vi "workbook add format.vi"(8 "error in (no error)":errorcluster, 11 "workbook":u32) -> (0 "error out":errorcluster, 3 "function return":u32)   [LabVIEW 8.6]
doc: "lxw_format workbook_add_format(lxw_workbook workbook);"
uses:
  pending_lvxlsxwriter/xlsxwriter.dll
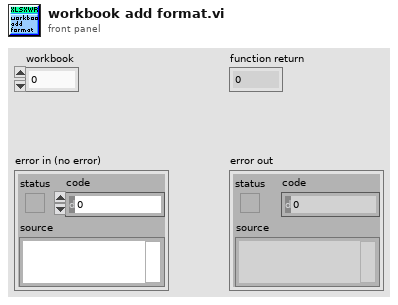
[diagram p1: front panel]
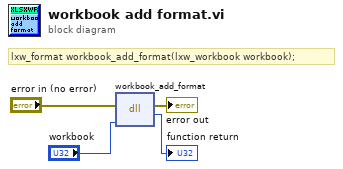
[diagram p0: block diagram]
diagram:
  # "lxw_format workbook_add_format(lxw_workbook workbook);"
  n1 = dll-call lib="C:/Users/WDAGUtilityAccount/Desktop/pending_lvxlsxwriter/xlsxwriter.*" fn="workbook_add_format"(error in="error in (no error)", "workbook"="workbook") -> (error out=→"error out":errorcluster, →"function return":u32)  [unwired: 3 in, 1 out]
